vi "ep_Speed Calculation Preprocess.vi"(10 "number of peaks":i32[](array[numeric]), 11 "enough points for peak search?":bool[](array[boolean])) -> (2 "harmonic for comparison":i32[](array[numeric]), 3 "case for speed calculation":T1)   [LabVIEW 2014, in "NI_EP_Motor Monitoring.lvlib"]
uses:
  <vilib>/addons/Electrical Power/Motor Monitoring/NI_EP_Motor Monitoring.lvlib
  <vilib>/addons/Electrical Power/Motor Monitoring/subVIs/ep_Case for Speed Calculation.ctl
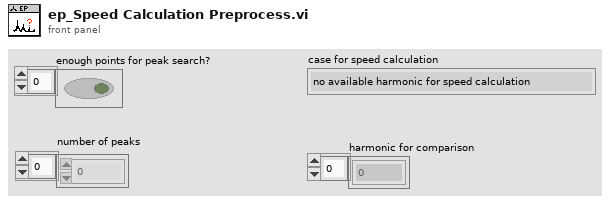
[diagram p1: front panel]
types:
  T1 = typedef "NI_EP_Motor Monitoring.lvlib/ep_Case for Speed Calculation.ctl" = enum16{"no available harmonic for speed calculation", "use the harmonic with highest magnitude", "use the harmonic with highest significance"}
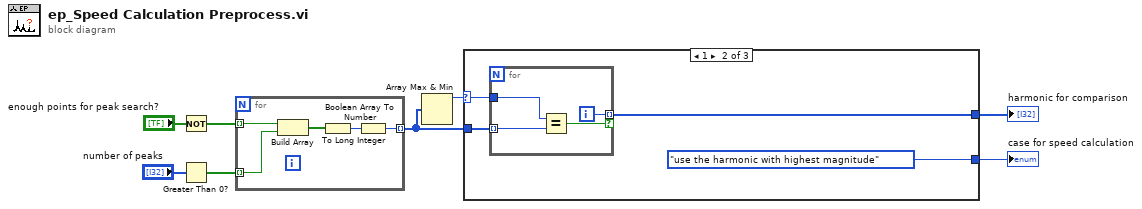
[diagram p0: block diagram]
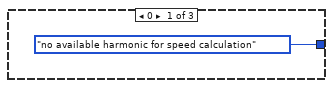
[diagram p2: hidden frame]
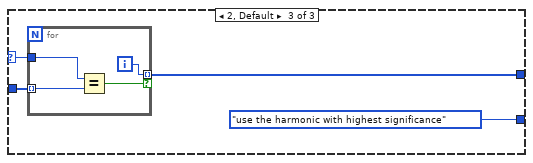
[diagram p3: hidden frame]
diagram:
  n1 = Not(x="enough points for peak search?") -> (.not. x?=w2:bool[])
  n2 = Greater Than 0?(x="number of peaks") -> (x > 0?=w1:bool[])
  n3 = for {
    tunnel: [w12] -> w7 mode=indexing
    tunnel: w2 -> [w10] mode=indexing
    tunnel: w1 -> [w9] mode=indexing
    n4 = Build Array(w10, w9) -> (w11:bool[])
    n5 = Boolean Array To Number(Boolean array=w11) -> (number=w13:u32)
    n6 = To Long Integer(number=w13) -> (32bit integer=w12:i32)
  }
  n7 = Array Max & Min(array=w7) -> (max value=w8:i32)  [unwired: 3 out]
  n8 = case shown="1" w8 {
    selector: w8 -> [_ w18 w26]
    tunnel: w7 -> [_ w17 w25]
    tunnel: [ep_Case_for_Speed_Calculation."no available harmonic for speed calculation" ("case for speed calculation") ep_Case_for_Speed_Calculation."use the harmonic with highest magnitude" ("case for speed calculation") ep_Case_for_Speed_Calculation."use the harmonic with highest significance" ("case for speed calculation")] -> w4
    tunnel: [_ w16 w24] -> w3
    frame 0 {
    }
    frame 1 {
      n9 = for {
        tunnel: w18 -> [w22]
        tunnel: w17 -> [w21] mode=indexing
        tunnel: [w20] -> w16 mode=indexing if=w19
        i -> [w20]
        n10 = Equal?(x=w22, y=w21) -> (x = y?=w19:bool)
      }
    }
    frame 2, Default {
      n11 = for {
        tunnel: w26 -> [w30]
        tunnel: w25 -> [w29] mode=indexing
        tunnel: [w28] -> w24 mode=indexing if=w27
        i -> [w28]
        n12 = Equal?(x=w30, y=w29) -> (x = y?=w27:bool)
      }
    }
  }
  "case for speed calculation" <- w4
  "harmonic for comparison" <- w3
